vi "Get Scanner Map.vi"(11 "Input":string[](array[string])) -> (3 "Scanners":T1(array[cluster]))   [LabVIEW 2021]
uses:
  <vilib>/regexp/Match Regular Expression.xnode
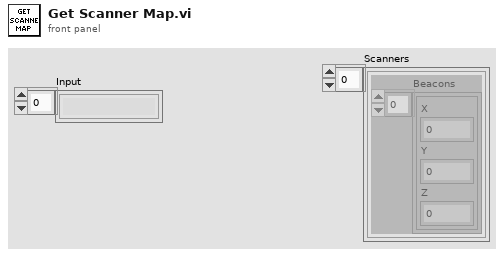
[diagram p1: front panel]
types:
  T1 = cluster{"Beacons":cluster{"X":i64, "Y":i64, "Z":i64}[]}[]
  T2 = cluster{"Beacons":cluster{"X":i64, "Y":i64, "Z":i64}[]}
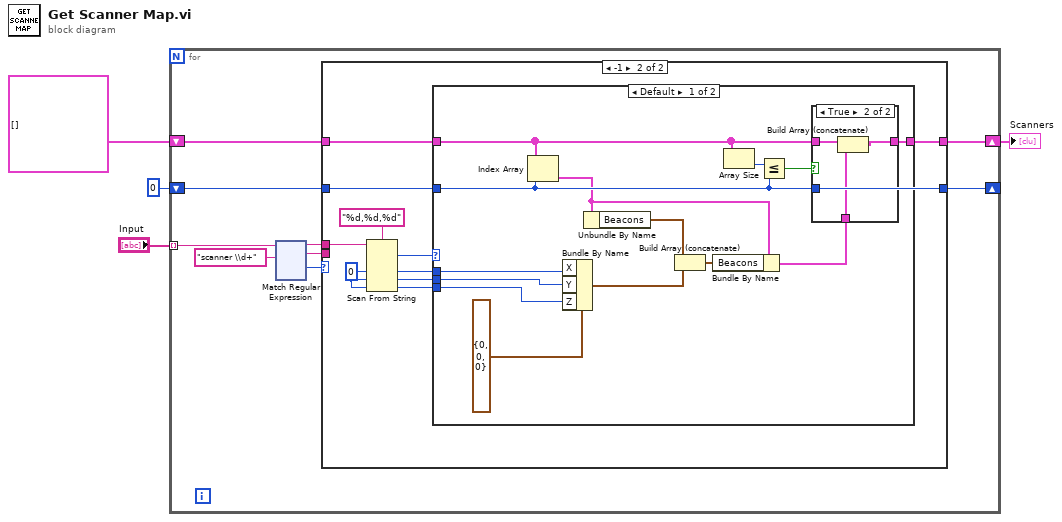
[diagram p0: block diagram]
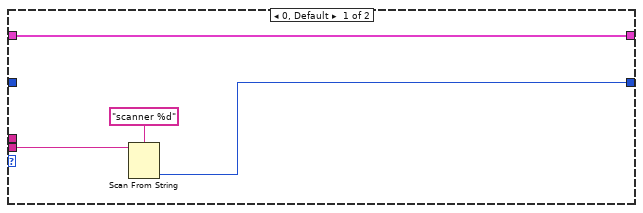
[diagram p2: hidden frame]
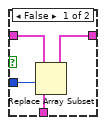
[diagram p3: hidden frame]
diagram:
  n1 = for {
    tunnel: "Input" -> [w13] mode=indexing
    shift-right: [w5] -> _
    shift-left: 0 -> [w10]
    shift-right: [w6] -> w1
    shift-left: T1 [] -> [w7]
    n2 = xnode "Match Regular Expression"("input string"=w13, "regular expression"="scanner \\d+") -> ("before match"=w8:string, "whole match"=w9:string, "offset past match"=w11:i32)  [unwired: 4 in, 2 out]
    n3 = case shown="-1" w11 {
      tunnel: w10 -> [_ w20]
      tunnel: w9 -> [w15 _]
      tunnel: [w16 w20] -> w5
      tunnel: w8 -> [_ w27]
      tunnel: w7 -> [w17 w22]
      tunnel: [w17 w21] -> w6
      frame 0, Default {
        n4 = Scan From String(format string="scanner %d", input string=w15) -> (output 1=w16:i32)  [unwired: 3 in, 3 out]
      }
      frame -1 {
        w18 = i64 0 ("default value 1")
        n5 = Scan From String(format string="%d,%d,%d", input string=w27, default 1=w18, default 2=w18, default 3=w18) -> (offset past scan=w19:u32, output 1=w25:i64, output 2=w24:i64, output 3=w23:i64)  [unwired: 2 in, 2 out]
        n6 = case shown="Default" w19 {
          tunnel: w25 -> [w38 _]
          tunnel: w24 -> [w37 _]
          tunnel: w23 -> [w36 _]
          tunnel: w22 -> [w34 w49]
          tunnel: [w41 w49] -> w21
          tunnel: w20 -> [w33 _]
          frame Default {
            n7 = Index Array(array=w34, index=w33) -> (element=w30:T2)
            n8 = Bundle By Name(cluster=cluster{"X":i64, "Y":i64, "Z":i64} {"X"=0, "Y"=0, "Z"=0}, "X"=w38, "Y"=w37, "Z"=w36) -> (w31:cluster{"X":i64, "Y":i64, "Z":i64})
            n9 = Unbundle By Name(w30) -> ("Beacons"=w32:cluster{"X":i64, "Y":i64, "Z":i64}[])
            n10 = Build Array (concatenate)(w32, w31) -> (w29:cluster{"X":i64, "Y":i64, "Z":i64}[])
            n11 = Bundle By Name(cluster=w30, "Beacons"=w29) -> (w28:T2)
            n12 = Array Size(array=w34) -> (size(s)=w40:i32)
            n13 = Less Or Equal?(x=w40, y=w33) -> (x <= y?=w39:bool)
            n14 = case shown="True" w39 {
              tunnel: [w45 w47] -> w41
              tunnel: w28 -> [w44 w46]
              tunnel: w34 -> [w43 w48]
              tunnel: w33 -> [w42 _]
              frame False {
                n15 = Replace Array Subset(array=w43, new element=w44, index=w42) -> (w45:T1)
              }
              frame True {
                n16 = Build Array (concatenate)(w48, w46) -> (w47:T1)
              }
            }
          }
          frame 0 {
          }
        }
      }
    }
  }
  "Scanners" <- w1
